vi "Single-Carrier Modulation.vi"(6 "Symbol Rate":i32=1, 7 "QAM Comparison":enum16{"MT Modulate", "Homebrew"}(ring), 8 "Sampling Rate":i32=10, 9 "frequency":dbl=1.0 format="%0.2p", 10 "DataLen":i32=512, 11 "QAM Complexity":T2(ring)) -> (1 "sampling info":cluster{"Fs":dbl, "#s":dbl}={"Fs"=1000.0, "#s"=1000.0} {"Fs" format="%.2p"}, 3 "waveform":waveform(cdb))   [LabVIEW 2018]
uses:
  <vilib>/measure/maspectr.llb/FFT Spectrum (Real-Im) for 1 Chan (CDB).vi
  <vilib>/measure/NI_MAPro.lvlib
  <vilib>/measure/NI_MABase.lvlib
panel:
  out "#s":dbl
  out "FFT Plot (Imaginary)":dbl[](graph)
  out "Constellation Graph":T1(graph)
  out "FFT Plot (Real)":waveform(dbl)(graph)
  out "Waveform Graph":i32[](graph)
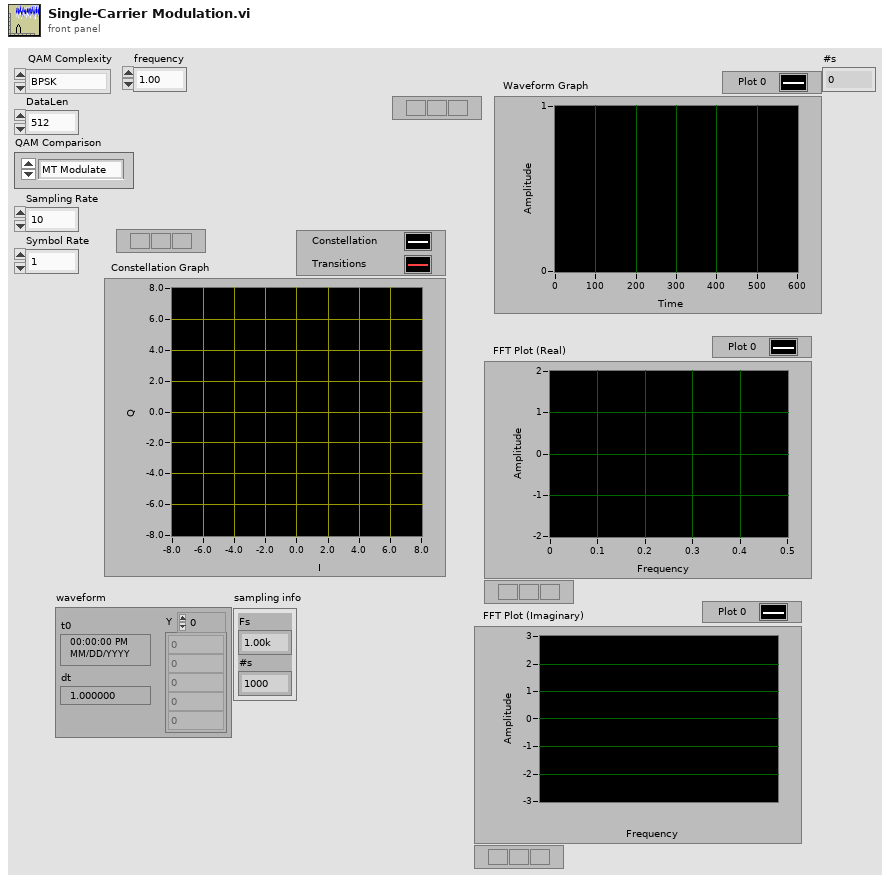
[diagram p1: front panel]
types:
  T1 = cluster{"Decimated Array":dbl[], "Decimated Array":dbl[]}[]
  T2 = enum16{"BPSK", "QPSK", "16-QAM", "64-QAM", "256-QAM"}
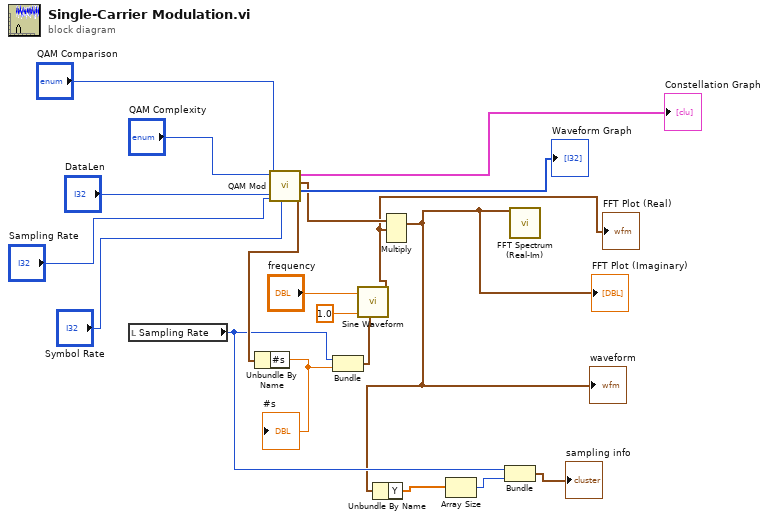
[diagram p0: block diagram]
diagram:
  n1 = local read "Sampling Rate"() -> (w8:i32)
  n2 = call "QAM Mod.vi"("Symbol Rate"="Symbol Rate", "Samples/Symbol"="Sampling Rate", "DataLen"="DataLen", "QAM Comparison"="QAM Comparison", "QAM Complexity"="QAM Complexity") -> ("sampling info"=w13:cluster{"Fs":dbl, "#s":dbl}, "Bitstream (Reference)"=→"Waveform Graph":i32[], "Waveform"=w5:waveform(cdb), "Constellation Graph"=→"Constellation Graph":T1)  [unwired: 1 out]
  n3 = Unbundle By Name(w13) -> ("#s"=w12:dbl)
  "#s" <- w12
  n4 = Bundle("Sampling Rate"=w8, "#s"=w12) -> (w9:cluster{"Sampling Rate":i32, "#s":dbl})  [unwired: 1 in]
  n5 = call <vilib>:"Sine Waveform.vi"("sampling info"=w9, "amplitude"=1.0, "frequency"="frequency") -> ("signal out"=w4:waveform(dbl))  [unwired: 7 in, 1 out]
  "FFT Plot (Real)" <- w4
  n6 = Multiply(1:w4, 2:w5) -> (0:w2:waveform(cdb))  [unwired: 1 in, 1 out]
  "FFT Plot (Imaginary)" <- w2
  "waveform" <- w2
  n7 = Unbundle By Name(w2) -> ("Y"=w3:cdb[])
  n8 = Array Size(array=w3) -> (size(s)=w7:i32)
  n9 = Bundle("Sampling Rate"=w8, w7) -> (→"sampling info":cluster{"Sampling Rate":i32, i32})  [unwired: 1 in]
  n10 = call-poly <vilib>:"FFT Spectrum (Real-Im).vi"("time signal"=w2) -> ()  [unwired: 6 in, 5 out]
